vi "SystemCore Get Team Number.vi"(11 "error in":errorcluster) -> (6 "Team Number":string, 15 "error out":errorcluster)   [LabVIEW 2026, in "MrcLib.lvlib"]
doc: "Returns the team number entered into the DS and robot controller."
uses:
  MrcLib.lvlib
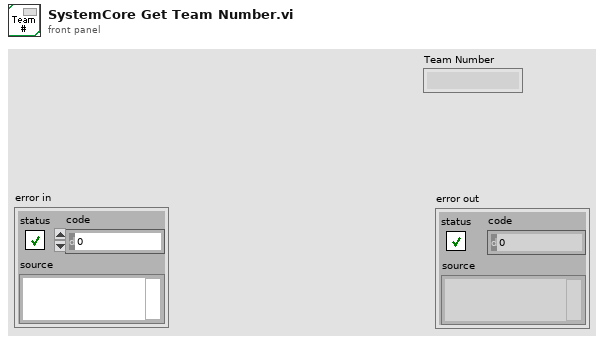
[diagram p1: front panel]
types:
  T1 = typedef "MRC String.ctl" = cluster{"pointer":u64, "length":u64}
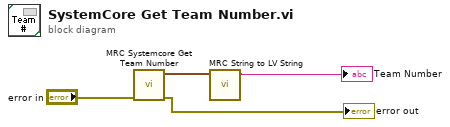
[diagram p0: block diagram]
diagram:
  n1 = call "MRC Systemcore Get Team Number.vi"("error in (no error)"="error in") -> ("error out"=→"error out":errorcluster, "team"=w4:T1)  [unwired: 9 in]
  n2 = call "MRC String to LV String.vi"("MRC String"=w4) -> ("LV String"=→"Team Number":string)  [unwired: 10 in]
